vi "TIMEGLOBAL.vi"() -> ()   [LabVIEW 2023]
panel:
  out "Timer Finished":bool
  out "Time Remaining":dbl
  in  "Start Time":dbl
  out "Time Elapsed":dbl
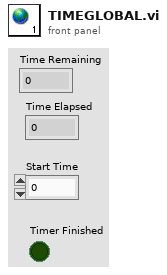
[diagram p1: front panel]
diagram:
